vi "Input String to Column Index.vi"(8 "error in (no error)":errorcluster, 10 "Input String":string, 11 "StateMachine in":refnum<class "StateMachine.lvclass">) -> (0 "error out":errorcluster, 1 "Column Index found?":bool, 2 "Column Index":i32)   [LabVIEW 2019, in "State Machine.lvlib" / "StateMachine.lvclass"]
uses:
  StateMachine.lvclass
  StateMachine.lvclass/StateMachine.ctl
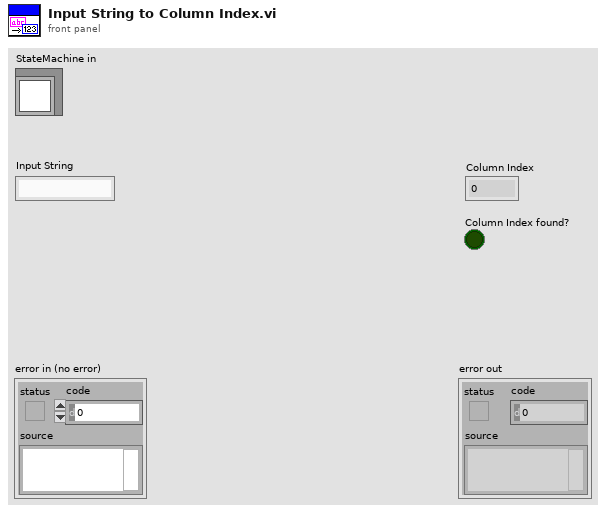
[diagram p1: front panel]
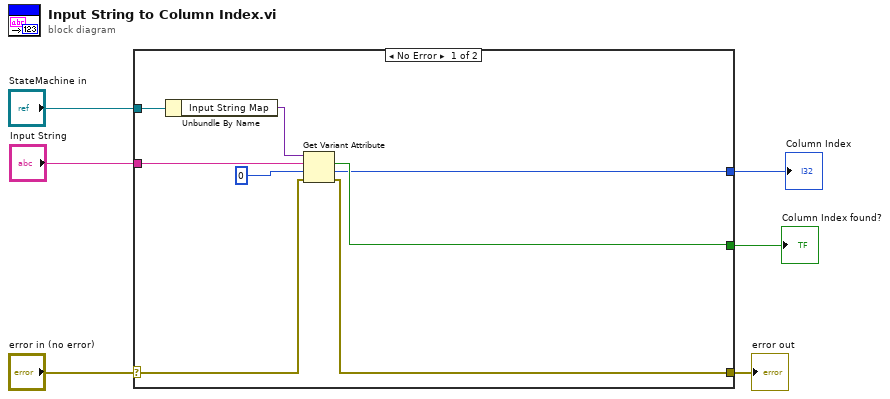
[diagram p0: block diagram]
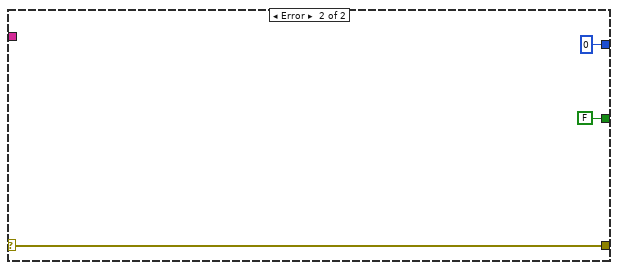
[diagram p2: hidden frame]
diagram:
  n1 = case shown="No Error" "error in (no error)" {
    selector: "error in (no error)" -> [w11 w17]
    tunnel: [w7 w17] -> w5
    tunnel: "StateMachine in" -> [w14 _]
    tunnel: "Input String" -> [w12 _]
    tunnel: [w10 FALSE] -> w1
    tunnel: [w8 0] -> w2
    frame No Error {
      n2 = Unbundle By Name(w14) -> ("Input String Map"=w13:variant)
      n3 = Get Variant Attribute(Variant=w13, name=w12, default value (empty Variant)=0, error in=w11) -> (found=w10:bool, value=w8:i32, error out=w7:errorcluster)  [unwired: 1 out]
    }
    frame Error {
    }
  }
  "error out" <- w5
  "Column Index" <- w2
  "Column Index found?" <- w1
